vi "Create Message Setter (from Template).vi"(8 "error in (no error)":errorcluster, 10 "RPC Message Name":string, 11 "RPC Messages Folder (ProjectItem) in":refnum<vi>) -> (0 "error out":errorcluster, 1 "Created?":bool, 2 "VI out":refnum<vi>, 3 "RPC Messages Folder (ProjectItem) out":refnum<vi>)   [LabVIEW 2019, in "gRPC Template Creation Utility.lvlib"]
uses:
  gRPC Template Creation Utility.lvlib
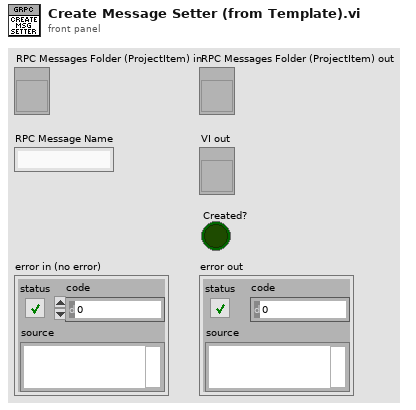
[diagram p1: front panel]
types:
  T1 = enum32{"invalid VI type", "Standard VI", "Control VI", "Global VI", "Polymorphic VI", "Configuration VI", "SubSystem", "Facade VI", "Method VI"}
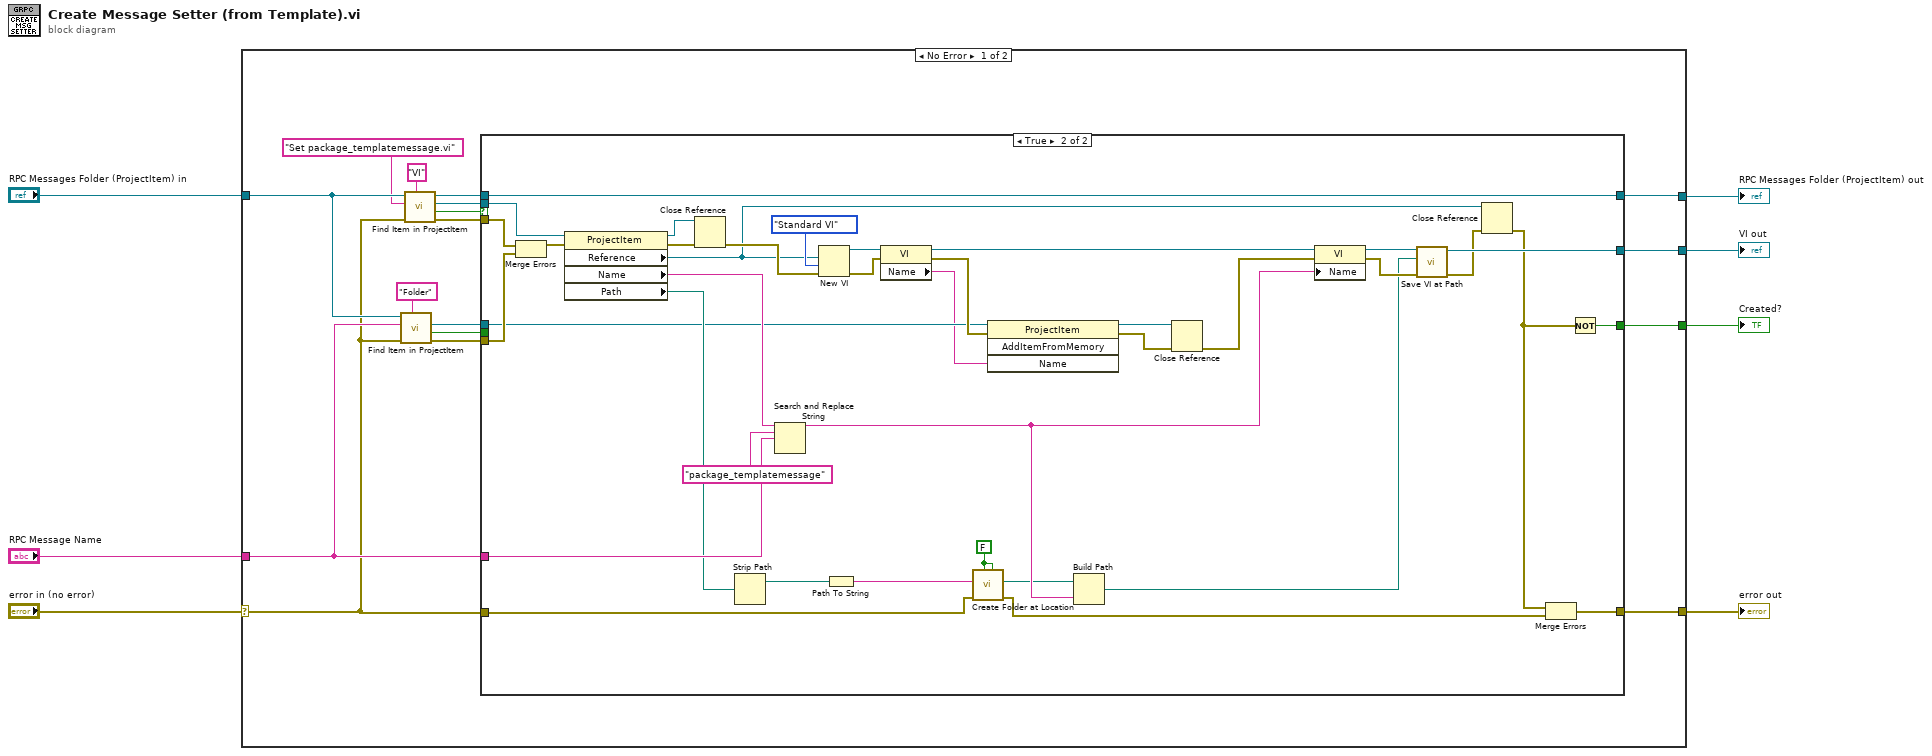
[diagram p0: block diagram]
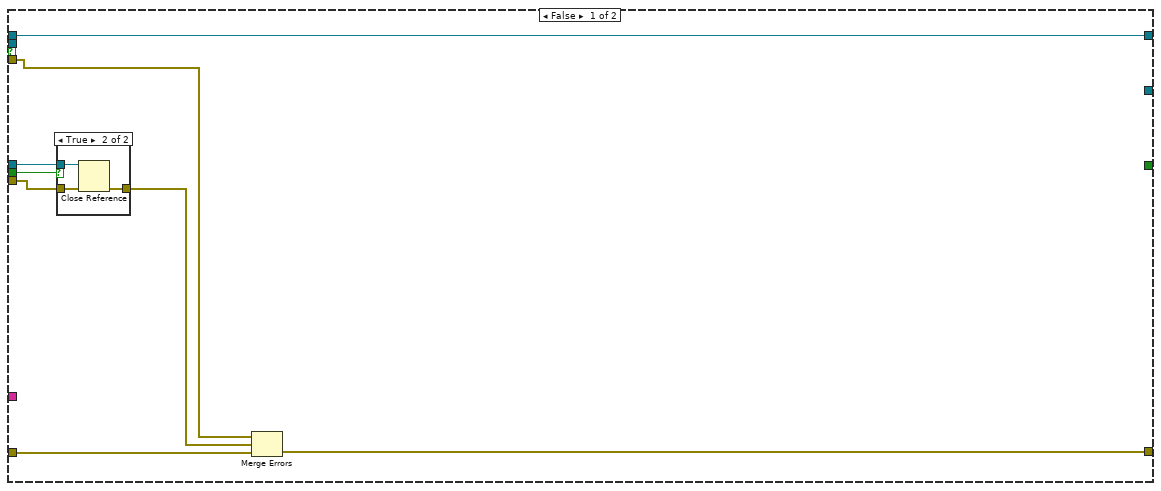
[diagram p2: hidden frame]
diagram:
  n1 = case shown="No Error" "error in (no error)" {
    selector: "error in (no error)" -> [w13 w75]
    tunnel: "RPC Message Name" -> [w24 _]
    tunnel: "RPC Messages Folder (ProjectItem) in" -> [w23 w76]
    tunnel: [w22 w75] -> w5
    tunnel: [w10 w76] -> w4
    tunnel: [w19 _] -> w3
    tunnel: [w9 _] -> w1
    frame No Error {
      n2 = call "Find Item in ProjectItem.vi"("Item Type"="Folder", "error in (no error)"=w13, "Name"=w24, "ProjectItem in"=w23) -> ("error out"=w21:errorcluster, "Found ?"=w8:bool, "Item Refnum out"=w18:refnum<vi>)  [unwired: 4 in, 1 out]
      n3 = call "Find Item in ProjectItem.vi"("Item Type"="VI", "error in (no error)"=w13, "Name"="Set package_templatemessage.vi", "ProjectItem in"=w23) -> ("error out"=w20:errorcluster, "Found ?"=w12:bool, "Item Refnum out"=w17:refnum<vi>, "ProjectItem out"=w11:refnum<vi>)  [unwired: 4 in]
      n4 = case shown="True" w12 {
        tunnel: w24 -> [_ w74]
        tunnel: [w27 w70] -> w22
        tunnel: w21 -> [w31 w68]
        tunnel: w20 -> [w26 w66]
        tunnel: [_ w64] -> w19
        tunnel: w18 -> [w30 w52]
        tunnel: w17 -> [_ w47]
        tunnel: w13 -> [w28 w46]
        tunnel: w11 -> [w32 w45]
        tunnel: [w32 w45] -> w10
        tunnel: [_ w41] -> w9
        tunnel: w8 -> [w25 _]
        frame False {
          n5 = case shown="True" w25 {
            tunnel: w31 -> [w33 w36]
            tunnel: w30 -> [_ w35]
            tunnel: [w33 w34] -> w29
            frame False {
            }
            frame True {
              n6 = Close Reference(reference=w35, error in (no error)=w36) -> (error out=w34:errorcluster)
            }
          }
          n7 = Merge Errors(w26, w29, w28) -> (w27:errorcluster)
        }
        frame True {
          w65 = FALSE ("Use Relative (F)")
          n8 = Merge Errors(w66, w68) -> (w67:errorcluster)
          n9 = property class="ProjectItem"(reference=w47, error in=w67) -> (reference out=w73:refnum<vi>, error out=w71:errorcluster, "Reference"=w38:refnum<vi>, "Name"=w56:string, "Path"=w54:path)
          n10 = Close Reference(reference=w73, error in (no error)=w71) -> (error out=w72:errorcluster)
          n11 = Strip Path(path=w54) -> (stripped path=w37:path)  [unwired: 1 out]
          n12 = Search and Replace String(input string=w56, search string="package_templatemessage", replace string=w74) -> (result string=w60:string)  [unwired: 5 in, 3 out]
          n13 = New VI(8:w72, 9:T1."Standard VI" ("vi type (standard vi)"), 10:w38) -> (0:w50:errorcluster, 3:w48:refnum<vi>)  [unwired: 1 in, 3 out]
          n14 = Path To String(path=w37) -> (string=w53:string)
          n15 = property class="VI"(reference=w48, error in=w50) -> (reference out=w57:refnum<vi>, error out=w58:errorcluster, "Name"=w51:string)
          n16 = call "Create Folder at Location.vi"("Override existing (F)"=w65, "Use Relative (F)"=w65, "Error In"=w46, "Path"=w53) -> ("Error Out"=w69:errorcluster, "Full path out"=w59:path)  [unwired: 5 in, 1 out]
          n17 = invoke class="ProjectItem" method="AddItemFromMemory"(reference=w52, error in=w58, "Name"=w51) -> (reference out=w43:refnum<vi>, error out=w44:errorcluster)  [unwired: 1 in, 2 out]
          n18 = Build Path(base path=w59, name or relative path=w60) -> (appended path=w62:path)
          n19 = Close Reference(reference=w43, error in (no error)=w44) -> (error out=w42:errorcluster)
          n20 = property class="VI"(reference=w57, error in=w42, "Name"=w60) -> (reference out=w61:refnum<vi>, error out=w63:errorcluster)
          n21 = call "Save VI at Path.vi"("error in (no error)"=w63, "Path"=w62, "VI in"=w61) -> ("error out"=w40:errorcluster, "VI out"=w64:refnum<vi>)  [unwired: 6 in, 1 out]
          n22 = Close Reference(reference=w38, error in (no error)=w40) -> (error out=w39:errorcluster)
          n23 = Merge Errors(w39, w69) -> (w70:errorcluster)
          n24 = Not(x=w39) -> (.not. x?=w41:bool)
        }
      }
    }
    frame Error {
    }
  }
  "error out" <- w5
  "RPC Messages Folder (ProjectItem) out" <- w4
  "VI out" <- w3
  "Created?" <- w1
